vi "config_AO_wav.vi"(5 "#s off":dbl, 6 "Channel config":T1={"Frequency"=10.0, "Voltage"=1.0, "Signal type"=enum."Sine Wave", "Square wave duty cycle (%)"=50.0, "physical channels"="", "name to assign"="", "Phase"=1.0, "Offset"=1.0} {"Square wave duty cycle (%)" format="%0.2f"}, 7 "Sampling info":cluster{"Fs":dbl, "#s":dbl}={"Fs"=1000.0, "#s"=1000.0} {"Fs" format="%.2p"}, 8 "error in":errorcluster, 11 "task in":refnum<k21>) -> (0 "error out":errorcluster, 3 "task out":refnum<k21>, 4 "AO Waveform Graph":waveform(dbl)(graph))   [LabVIEW 2019]
doc: "This example demonstrates how to acquire a continuous amount of data (Waveform) using the DAQ device's internal clock. It also shows how to synchronize two devices for different device families (E Series, S Series, M Series, X Series, DSA, and SC Express), to simultaneously acquire the data.\n\nFor instructions on how to connect your signals to the DAQ device, refer to your device documentation."
uses:
  <vilib>/DAQmx/write.llb/DAQmx Write (Analog Wfm 1Chan NSamp).vi
  <vilib>/DAQmx/create/channels.llb/DAQmx Create Channel (AO-Voltage-Basic).vi
  <vilib>/DAQmx/configure/timing.llb/DAQmx Timing (Sample Clock).vi
  <vilib>/DAQmx/miscellaneous.llb/DAQmx Fill In Error Info.vi
  <vilib>/Waveform/WDTOps.llb/WDT Append Waveforms DBL.vi
  <vilib>/measure/NI_MABase.lvlib
panel:
  # "Config AO - Waveform"
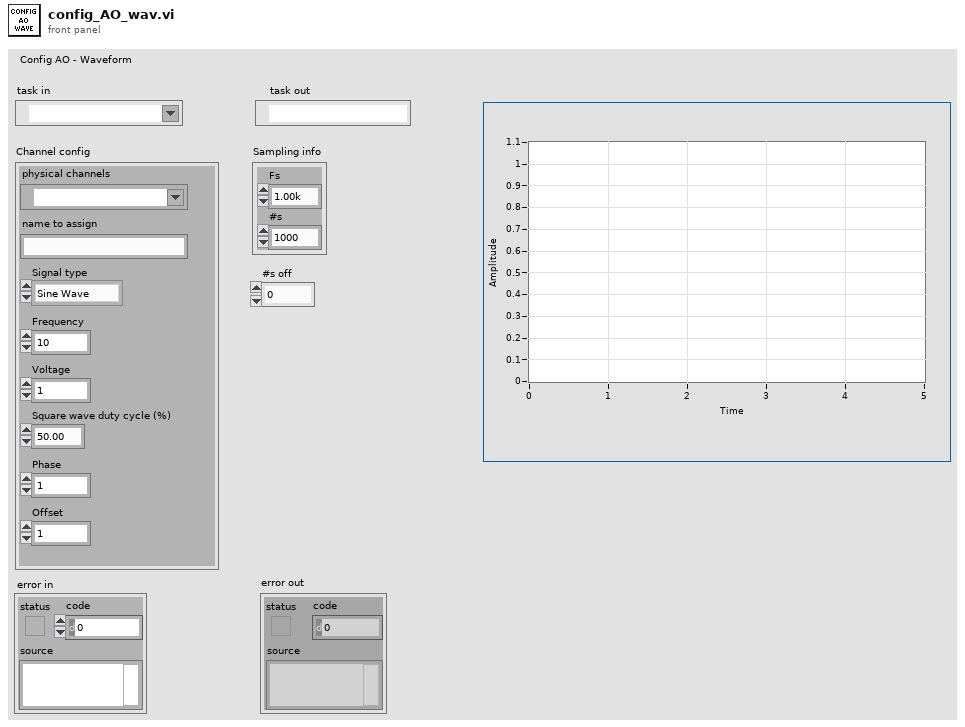
[diagram p1: front panel]
types:
  T1 = cluster{"Frequency":dbl, "Voltage":dbl, "Signal type":enum16{"Sine Wave", "Triangle Wave", "Square Wave", "Sawtooth Wave"}, "Square wave duty cycle (%)":dbl, "physical channels":tag, "name to assign":string, "Phase":dbl, "Offset":dbl}
  T2 = enum16{"Sine Wave", "Triangle Wave", "Square Wave", "Sawtooth Wave"}
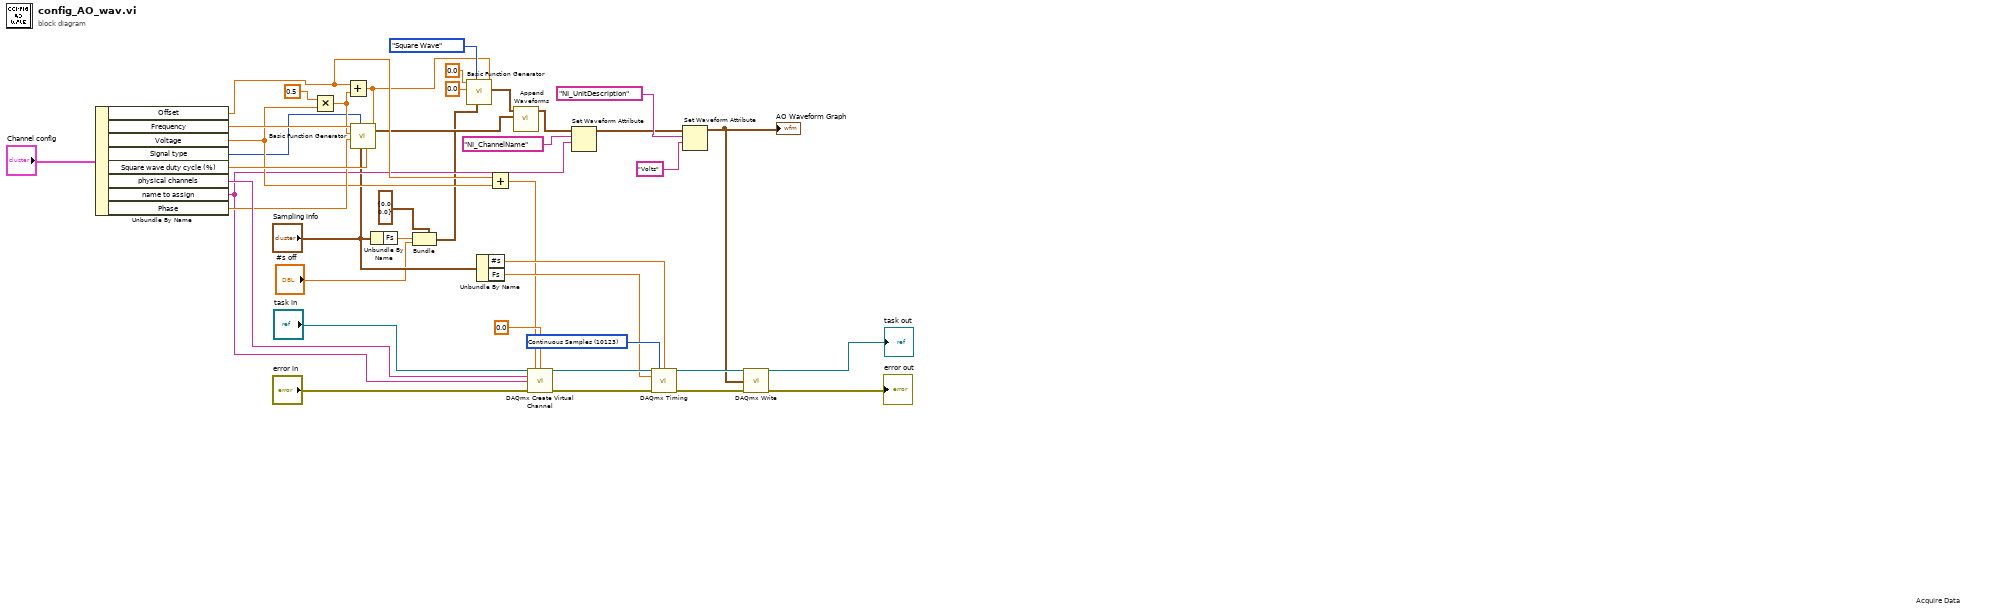
[diagram p0: block diagram]
diagram:
  w30 = 10123 items=["Finite Samples"=10178, "Continuous Samples"=10123, "Hardware Timed Single Point"=12522] ("sample mode")
  # "Acquire Data"
  n1 = Unbundle By Name("Channel config") -> ("Offset"=w21:dbl, "Frequency"=w36:dbl, "Voltage"=w22:dbl, "Signal type"=w11:T2, "Square wave duty cycle (%)"=w35:dbl, "physical channels"=w25:tag, "name to assign"=w14:string, "Phase"=w24:dbl)
  n2 = Multiply(x=0.5, y=w22) -> (x*y=w23:dbl)
  n3 = Add(x=w21, y=w23) -> (x+y=w1:dbl)
  n4 = call <vilib>:"Basic Function Generator.vi"("offset"=w1, "square wave duty cycle (%)"=w35, "sampling info"="Sampling info", "signal type"=w11, "phase"=w24, "amplitude"=w23, "frequency"=w36) -> ("signal out"=w10:waveform(dbl))  [unwired: 2 in, 2 out]
  n5 = Unbundle By Name("Sampling info") -> ("Fs"=w6:dbl)
  n6 = Bundle(cluster=cluster{"Fs":dbl, "#s":dbl} {"Fs"=0.0, "#s"=0.0} ("sampling info"), "Fs"=w6, "#s"="#s off") -> (w3:cluster{"Fs":dbl, "#s":dbl})
  n7 = call <vilib>:"Basic Function Generator.vi"("offset"=w1, "sampling info"=w3, "signal type"=T2."Square Wave", "amplitude"=0.0, "frequency"=0.0) -> ("signal out"=w9:waveform(dbl))  [unwired: 4 in, 2 out]
  n8 = Unbundle By Name("Sampling info") -> ("#s"=w29:dbl, "Fs"=w28:dbl)
  n9 = Add(x=w21, y=w22) -> (x+y=w20:dbl)
  n10 = call-poly <vilib>:"Append Waveforms.vi"("waveform B"=w10, "waveform A"=w9) -> ("waveform out"=w8:waveform(dbl))  [unwired: 8 in, 1 out]
  n11 = call-poly <vilib>:"DAQmx Create Virtual Channel.vi"("task in"="task in", "maximum value"=w20, "minimum value"=0.0, "physical channels"=w25, "name to assign"=w14, "error in"="error in") -> ("task out"=w34:refnum<k21>, "error out"=w33:errorcluster)  [unwired: 8 in]
  n12 = Set Waveform Attribute(5:w14, 6:"NI_ChannelName" ("name"), 7:w8) -> (3:w17:waveform(dbl))  [unwired: 1 in, 2 out]
  n13 = call-poly <vilib>:"DAQmx Timing.vi"("task/channels in"=w34, "sample mode"=w30, "samples per channel"=w29, "rate"=w28, "error in"=w33) -> ("task out"=w31:refnum<k21>, "error out"=w32:errorcluster)  [unwired: 9 in]
  n14 = Set Waveform Attribute(5:"Volts" ("name"), 6:"NI_UnitDescription" ("name"), 7:w17) -> (3:w15:waveform(dbl))  [unwired: 1 in, 2 out]
  "AO Waveform Graph" <- w15
  n15 = call-poly <vilib>:"DAQmx Write.vi"("task/channels in"=w31, "data"=w15, "error in"=w32) -> ("task out"=→"task out":refnum<k21>, "error out"=→"error out":errorcluster)  [unwired: 10 in, 1 out]
